vi "DSF.Engine.Memory.Cache.Max Channel Count.vi"(8 "error in (no error)":errorcluster, 11 "Cache in":refnum<class "DSF.Engine.Memory.Cache.lvclass">) -> (0 "error out":errorcluster, 2 "max channel count":u64, 3 "Cache out":refnum<class "DSF.Engine.Memory.Cache.lvclass">)   [LabVIEW 2017, in "DSF.Engine.lvlib" / "DSF.Engine.Memory.Cache.lvclass"]
uses:
  DSF.Engine.Memory.Cache.lvclass
  DSF.Engine.Memory.Cache.lvclass/DSF.Engine.Memory.Cache.ctl
  Transfer/DSF.Engine.Transfer Group.lvclass
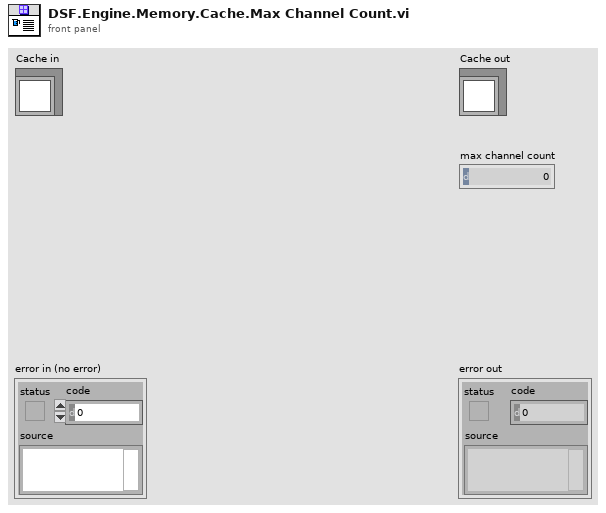
[diagram p1: front panel]
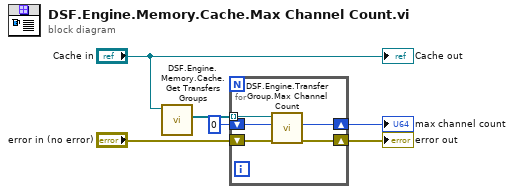
[diagram p0: block diagram]
diagram:
  n1 = call "DSF.Engine.Memory.Cache.Get Transfers Groups.vi"("Cache in"="Cache in") -> ("Transfers Groups"=w5:refnum<class "DSF.Engine.Transfer Group.lvclass">[])  [unwired: 9 in, 1 out]
  n2 = for {
    tunnel: w5 -> [w11] mode=indexing
    shift-right: [w7] -> w3
    shift-left: u64 0 ("max channel count") -> [w10]
    shift-right: [w8] -> w1
    shift-left: "error in (no error)" -> [w9]
    n3 = call "DSF.Engine.Transfer Group.Max Channel Count.vi"("error in (no error)"=w9, "max count in (0)"=w10, "Transfer Group in"=w11) -> ("error out"=w8:errorcluster, "max count out"=w7:u64)  [unwired: 6 in, 1 out]
  }
  "error out" <- w1
  "max channel count" <- w3
  "Cache out" <- "Cache in"
